vi "Default Plugin Subpanel.vi"() -> ()   [LabVIEW 2021, in "CIF Manager UI.lvlib"]
uses:
  CIF Manager UI.lvlib
  <vilib>/CIF Foundation/CIF Core/CIFUI/Typedef/Class Data for SubPanel.ctl
  <vilib>/CIF Foundation/CIF Core/CIFUI/Typedef/Core UI References.ctl
  <vilib>/CIF Foundation/CIF Core/CIFUI/Typedef/Run Listen Button.ctl
  <vilib>/CIF Foundation/CIF Core/CIFUI/Typedef/SubPanel Events.ctl
  <vilib>/CIF Foundation/CIF Core/CIFUI/Typedef/New Connection Plugin Event Data.ctl
  <vilib>/CIF Foundation/CIF Core/CIFUI/CIF_UI.lvclass
  <vilib>/CIF Foundation/CIF Core/CIFUI/CIF_UI.lvclass/CIF_UI.ctl
  <vilib>/CIF Foundation/CIF Core/CIFUI/Utilities/Get Human Readable Error.vi
  <vilib>/CIF Foundation/CIF Utilities/Errors/Append Error Location.vi
  <vilib>/CIF Foundation/CIF Utilities/Errors/Human Readable Error Message.vi
  <vilib>/CIF Foundation/CIF Core/CIFCore/Grpc/CIFCoreWrapper/CIFCoreWrapper.lvlib
panel:
  in  "Update Config":bool
  in  "Class Data for SubPanel":T1
  in  "New Config":string
  out "Current Config":string
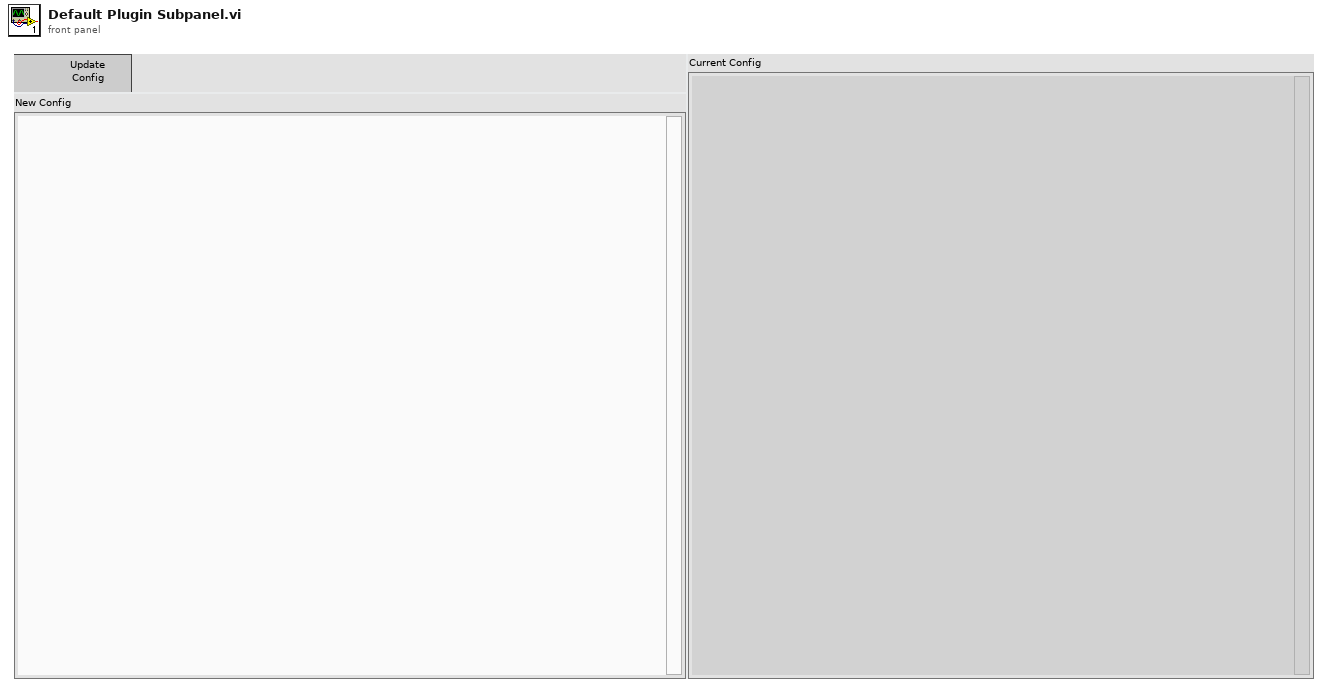
[diagram p1: front panel]
types:
  T1 = typedef "CIF_UI.lvclass/Class Data for SubPanel.ctl" = cluster{"IP Address":string, "Server Certificate File (.crt)":path, "Connected":bool, "Core UI References":T2, "Subpanel Events":T3}
  T2 = typedef "CIF_UI.lvclass/Core UI References.ctl" = cluster{"Plugin Status":refnum<vi>, "Plugin Status Valid":bool, "Connection":refnum<vi>, "Connection Valid":bool, "Exit":refnum<vi>, "Exit Valid":bool, "Run Listen":refnum<vi>, "Run Listen Valid":bool, "Clear Local Error":refnum<vi>, "Clear Local Error Valid":bool, "Local Error":refnum<vi>, "Local Error Valid":bool}
  T3 = typedef "CIF_UI.lvclass/SubPanel Events.ctl" = cluster{"Clear Local Error":refnum<user-event>, "Shutdown":refnum<user-event>, "Plugin Connection":refnum<user-event>}
  T4 = typedef "grpc-lvsupport-release.lvlib/grpcId.ctl" = u64
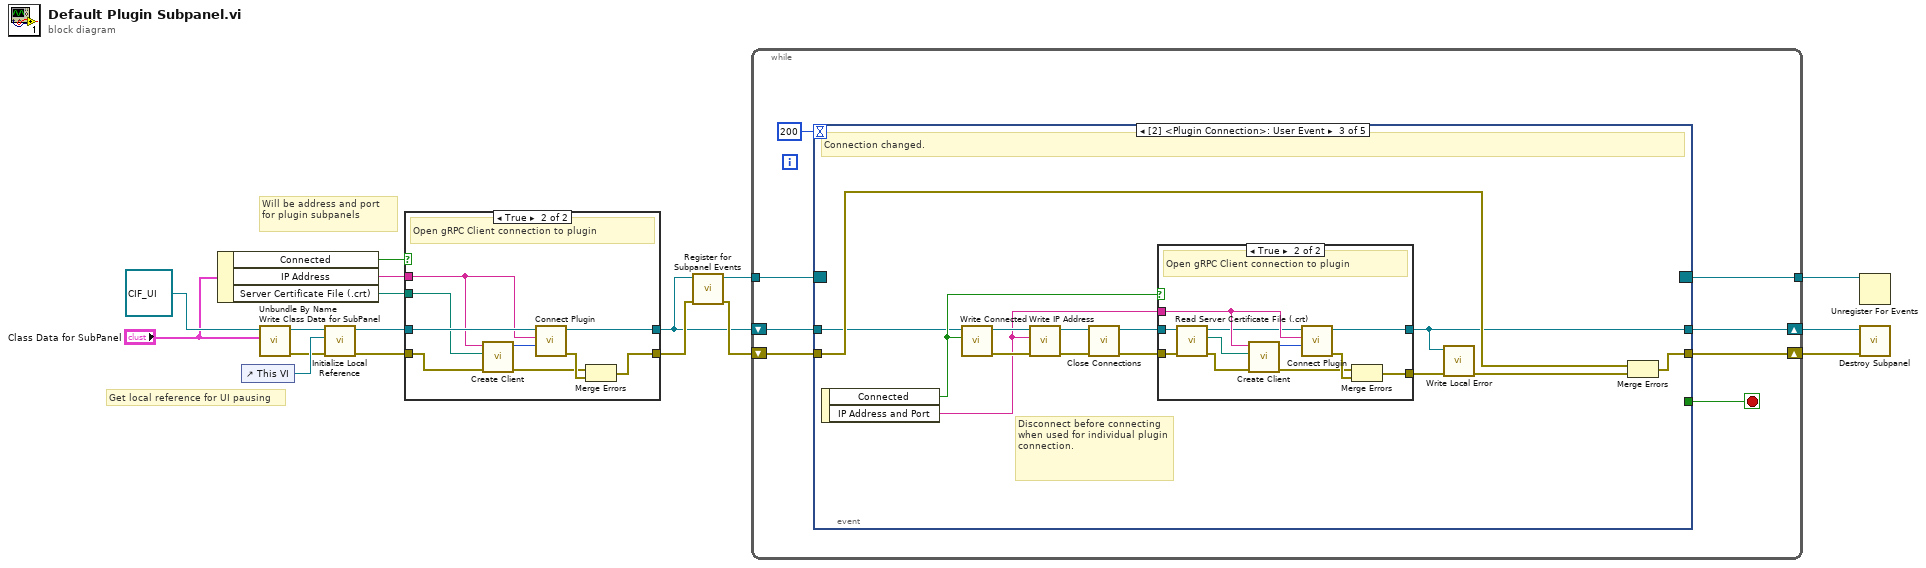
[diagram p0: block diagram]
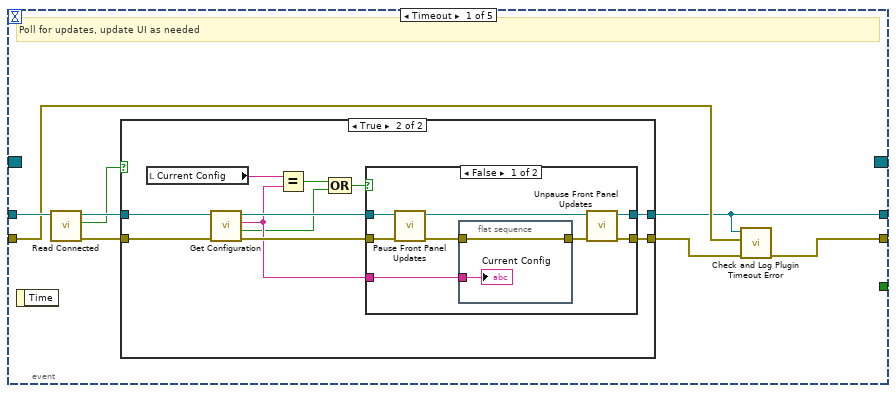
[diagram p3: hidden frame]
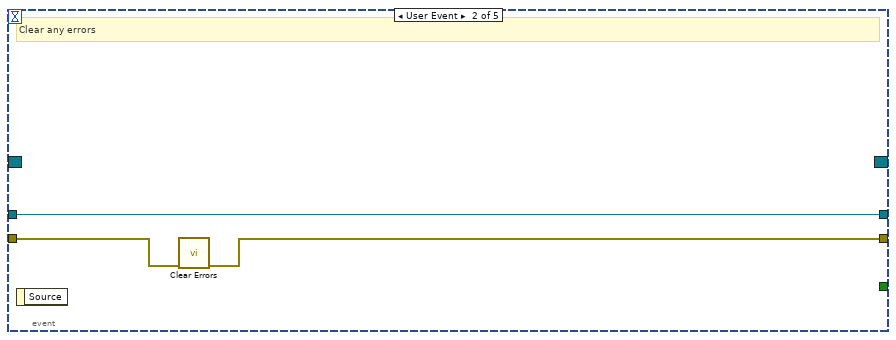
[diagram p6: hidden frame]
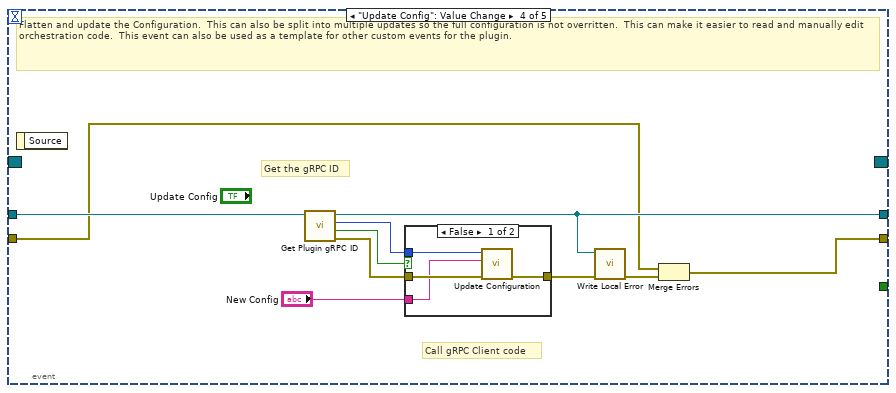
[diagram p8: hidden frame]
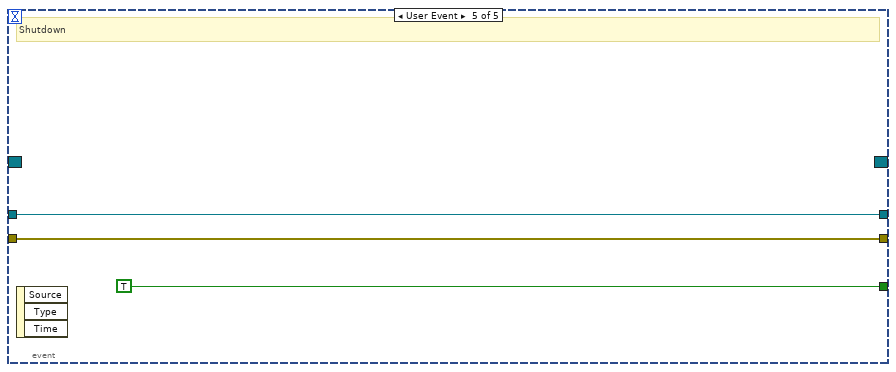
[diagram p10: hidden frame]
diagram:
  # "Will be address and port for plugin subpanels"
  # "Get local reference for UI pausing"
  n1 = Unbundle By Name("Class Data for SubPanel") -> ("Connected"=w8:bool, "IP Address"=w7:string, "Server Certificate File (.crt)"=w6:path)
  n2 = control-ref of="This VI"() -> (w17:refnum<vi>)
  n3 = call <vilib>:"Write Class Data for SubPanel.vi"("Class Data for SubPanel"="Class Data for SubPanel", "CIF_UI in"=refnum<class "CIF_UI.lvclass"> refnum) -> ("error out"=w12:errorcluster, "CIF_UI out"=w14:refnum<class "CIF_UI.lvclass">)  [unwired: 8 in]
  n4 = call <vilib>:"Initialize Local Reference.vi"("error in (no error)"=w12, "This VI"=w17, "CIF_UI in"=w14) -> ("error out"=w10:errorcluster, "CIF_UI out"=w11:refnum<class "CIF_UI.lvclass">)  [unwired: 7 in]
  n5 = case shown="True" w8 {
    tunnel: [w18 w28] -> w4
    tunnel: [w19 w26] -> w2
    tunnel: w11 -> [w19 w25]
    tunnel: w10 -> [w18 w24]
    tunnel: w7 -> [_ w21]
    tunnel: w6 -> [_ w20]
    frame False {
    }
    frame True {
      # "Open gRPC Client connection to plugin"
      n6 = call <vilib>:"Create Client.vi"("error in"=w24, "Server Certificate File (.crt)"=w20, "address"=w21) -> ("error out"=w23:errorcluster, "gRPC ID Out"=w22:T4)  [unwired: 7 in]
      n7 = call <vilib>:"Connect Plugin.vi"("gRPC ID"=w22, "Address"=w21, "CIF_UI in"=w25) -> ("error out"=w27:errorcluster, "CIF_UI out"=w26:refnum<class "CIF_UI.lvclass">)  [unwired: 7 in]
      n8 = Merge Errors(w23, w27) -> (w28:errorcluster)
    }
  }
  n9 = call <vilib>:"Register for Subpanel Events.vi"("error in (no error)"=w4, "CIF_UI in"=w2) -> ("error out"=w3:errorcluster, "Event Registration Refnum"=w1:refnum<event-registration>)  [unwired: 8 in]
  n10 = while {
    tunnel: w1 -> [w29]
    shift-right: [w31] -> w16
    shift-left: w2 -> [w34]
    shift-right: [w32] -> w5
    shift-left: w3 -> [w33]
    tunnel: [w30] -> w15
    stop <- w35 stop-if-true
    n11 = event shown="[2] <Plugin Connection>: User Event" {
      selector: w29 -> [_ _ _ _ _]
      dyn-events: [_ _ _ _ _] -> w30
      timeout: 200 -> [_ _ _ _ _]
      tunnel: [_ _ _ _ TRUE] -> w35
      tunnel: w34 -> [w41 w70 w73 w106 w116]
      tunnel: w33 -> [w38 w72 w76 w101 w115]
      tunnel: [w40 w71 w75 w100 w115] -> w32
      tunnel: [w37 w70 w74 w105 w116] -> w31
      event Timeout {
        # "Poll for updates, update UI as needed"
        n12 = event-data() -> ()  [unwired: 1 in, 1 out]
        n13 = call <vilib>:"Read Connected.vi"("CIF_UI in"=w41) -> ("error out"=w43:errorcluster, "Connected"=w42:bool, "CIF_UI out"=w44:refnum<class "CIF_UI.lvclass">)  [unwired: 8 in]
        n14 = case shown="True" w42 {
          tunnel: w43 -> [w45 w54]
          tunnel: [w45 w57] -> w39
          tunnel: w44 -> [w46 w55]
          tunnel: [w46 w56] -> w37
          frame False {
          }
          frame True {
            n15 = local read "Current Config"() -> (w51:string)
            n16 = call <vilib>:"Get Configuration.vi"("error in (no error)"=w54, "CIF_Plugin_UI in"=w55) -> ("error out"=w52:errorcluster, "Not Found"=w48:bool, "JSON Configuration"=w50:string, "CIF_Plugin_UI out"=w53:refnum<class "CIF_UI.lvclass">)  [unwired: 6 in]
            n17 = Equal?(x=w51, y=w50) -> (x = y?=w49:bool)
            n18 = Compound Arithmetic op=OR(w49, w48) -> (w47:bool)
            n19 = case shown="False" w47 {
              tunnel: [w65 w68] -> w57
              tunnel: [w64 w69] -> w56
              tunnel: w53 -> [w63 w69]
              tunnel: w52 -> [w62 w68]
              tunnel: w50 -> [w58 _]
              frame False {
                n20 = call <vilib>:"Pause Front Panel Updates.vi"("error in (no error)"=w62, "CIF_UI in"=w63) -> ("error out"=w60:errorcluster, "CIF_UI out"=w61:refnum<class "CIF_UI.lvclass">)  [unwired: 8 in]
                n21 = flat-sequence {
                  tunnel: w60 -> [w67]
                  tunnel: [w67] -> w59
                  tunnel: w58 -> [w66]
                  frame #0 {
                    "Current Config" <- w66
                  }
                }
                n22 = call <vilib>:"Unpause Front Panel Updates.vi"("error in (no error)"=w59, "CIF_UI in"=w61) -> ("error out"=w65:errorcluster, "CIF_UI out"=w64:refnum<class "CIF_UI.lvclass">)  [unwired: 8 in]
              }
              frame True {
              }
            }
          }
        }
        n23 = call <vilib>:"Check and Log Plugin Timeout Error.vi"("New Error"=w39, "Previous Error"=w38, "CIF_UI in"=w37) -> ("error out"=w40:errorcluster)  [unwired: 8 in]
      }
      event User Event {
        # "Clear any errors"
        n24 = event-data() -> ()  [unwired: 1 in, 1 out]
        n25 = call <vilib>:"Clear Errors.vi"("error in (no error)"=w72) -> ("error out"=w71:errorcluster)  [unwired: 5 in, 1 out]
      }
      event User Event {
        # "Disconnect before connecting when used for individual plugin connection."
        # "Connection changed."
        n26 = event-data() -> ("Connected"=w79:bool, "IP Address and Port"=w80:string)  [unwired: 1 in]
        n27 = call <vilib>:"Write Connected.vi"("Connected"=w79, "CIF_UI in"=w73) -> ("error out"=w85:errorcluster, "CIF_UI out"=w86:refnum<class "CIF_UI.lvclass">)  [unwired: 8 in]
        n28 = call <vilib>:"Write IP Address.vi"("error in (no error)"=w85, "IP Address"=w80, "CIF_UI in"=w86) -> ("error out"=w83:errorcluster, "CIF_UI out"=w84:refnum<class "CIF_UI.lvclass">)  [unwired: 7 in]
        n29 = call <vilib>:"Close Connections.vi"("error in (no error)"=w83, "CIF_UI in"=w84) -> ("error out"=w81:errorcluster, "CIF_UI out"=w82:refnum<class "CIF_UI.lvclass">)  [unwired: 8 in]
        n30 = case shown="True" w79 {
          tunnel: [w87 w99] -> w78
          tunnel: [w88 w97] -> w74
          tunnel: w82 -> [w88 w93]
          tunnel: w81 -> [w87 w92]
          tunnel: w80 -> [_ w94]
          frame False {
          }
          frame True {
            # "Open gRPC Client connection to plugin"
            n31 = call <vilib>:"Read Server Certificate File (.crt).vi"("error in (no error)"=w92, "CIF_UI in"=w93) -> ("error out"=w90:errorcluster, "Server Certificate File (.crt)"=w89:path, "CIF_UI out"=w91:refnum<class "CIF_UI.lvclass">)  [unwired: 7 in]
            n32 = call <vilib>:"Create Client.vi"("error in"=w90, "Server Certificate File (.crt)"=w89, "address"=w94) -> ("error out"=w96:errorcluster, "gRPC ID Out"=w95:T4)  [unwired: 7 in]
            n33 = call <vilib>:"Connect Plugin.vi"("gRPC ID"=w95, "Address"=w94, "CIF_UI in"=w91) -> ("error out"=w98:errorcluster, "CIF_UI out"=w97:refnum<class "CIF_UI.lvclass">)  [unwired: 7 in]
            n34 = Merge Errors(w96, w98) -> (w99:errorcluster)
          }
        }
        n35 = call <vilib>:"Write Local Error.vi"("error in (no error)"=w78, "CIF_UI in"=w74) -> ("error out"=w77:errorcluster)  [unwired: 9 in]
        n36 = Merge Errors(w76, w77) -> (w75:errorcluster)
      }
      event "Update Config": Value Change {
        # "Call gRPC Client code"
        # "Get the gRPC ID"
        # "Flatten and update the Configuration.  This can also be split into multiple updates so the full configuration is not overritten.  This can make it easier to read and manually edit orchestration code.  This event can also be used as a template for other custom events for the plugin."
        n37 = event-data() -> ()  [unwired: 1 in, 1 out]
        n38 = call <vilib>:"Get Plugin gRPC ID.vi"("CIF_UI in"=w106) -> ("error out"=w107:errorcluster, "Not Found"=w108:bool, "gRPC ID"=w109:T4, "CIF_UI out"=w105:refnum<class "CIF_UI.lvclass">)  [unwired: 6 in, 1 out]
        n39 = case shown="False" w108 {
          tunnel: w109 -> [w113 _]
          tunnel: w107 -> [w112 w114]
          tunnel: [w111 w114] -> w104
          tunnel: "New Config" -> [w110 _]
          frame False {
            n40 = call <vilib>:"Update Configuration.vi"("error in"=w112, "JSON Configuration"=w110, "gRPC ID"=w113) -> ("error out"=w111:errorcluster)  [unwired: 7 in, 1 out]
          }
          frame True {
          }
        }
        n41 = call <vilib>:"Write Local Error.vi"("error in (no error)"=w104, "CIF_UI in"=w105) -> ("error out"=w102:errorcluster)  [unwired: 9 in]
        n42 = Merge Errors(w101, w102) -> (w100:errorcluster)
      }
      event User Event {
        # "Shutdown"
        n43 = event-data() -> ()  [unwired: 1 in, 3 out]
      }
    }
  }
  n44 = Unregister For Events(event registration refnum=w15) -> ()  [unwired: 1 in, 1 out]
  n45 = call <vilib>:"Destroy Subpanel.vi"("error in (no error)"=w5, "CIF_UI in"=w16) -> ()  [unwired: 8 in, 2 out]
